vi "Create Server.vi"(5 "Server Key File (.key)":path, 7 "Server Certificate File (.crt)":path, 8 "error in":errorcluster, 11 "Server Address":string) -> (0 "error out":errorcluster, 3 "gRPC server out":refnum<class "Servicer.lvclass">)   [LabVIEW 2019, in "gRPC-servicer.lvlib" / "Servicer.lvclass"]
uses:
  Servicer.lvclass
  gRPC lv Support/grpc-lvsupport.lvlib
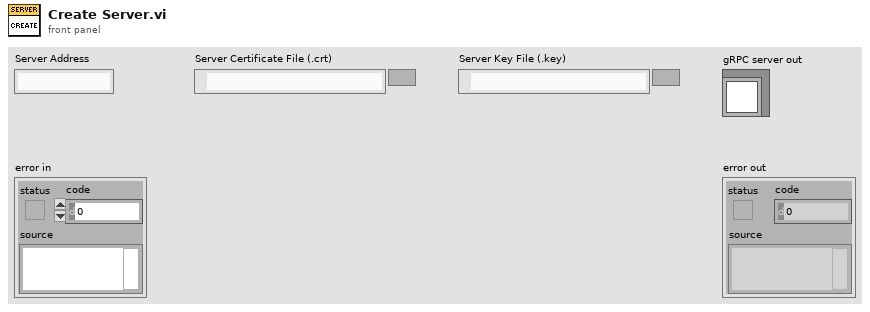
[diagram p1: front panel]
types:
  T1 = typedef "grpc-lvsupport.lvlib/grpcId.ctl" = u64
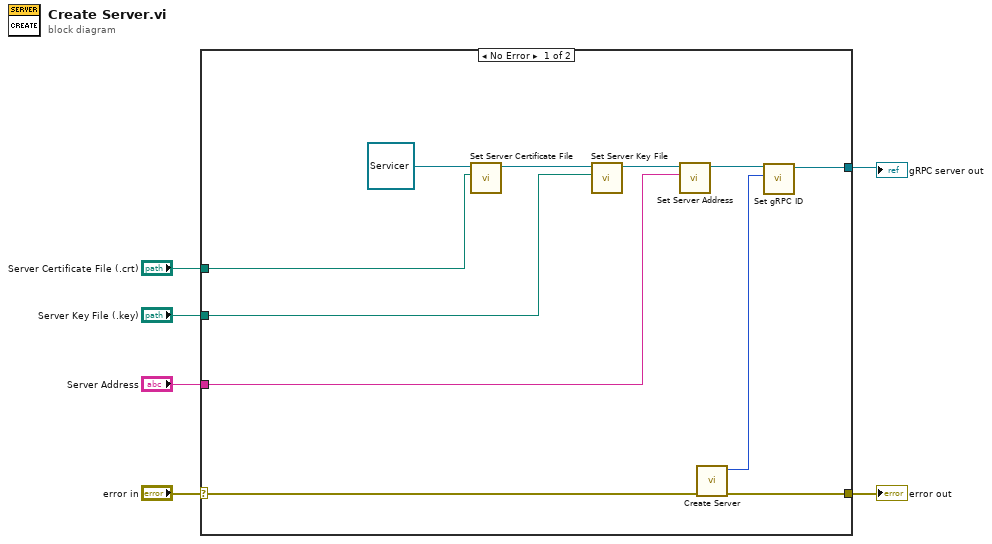
[diagram p0: block diagram]
diagram:
  n1 = case shown="No Error" "error in" {
    selector: "error in" -> [w17 w18]
    tunnel: [w16 w18] -> w5
    tunnel: [w7 _] -> w4
    tunnel: "Server Certificate File (.crt)" -> [w11 _]
    tunnel: "Server Key File (.key)" -> [w10 _]
    tunnel: "Server Address" -> [w9 _]
    frame No Error {
      n2 = call "Set Server Certificate File.vi"("Server Certificate File (.crt)"=w11, "gRPC server in"=refnum<class "Servicer.lvclass"> refnum ("OOP Server out")) -> ("gRPC server out"=w14:refnum<class "Servicer.lvclass">)  [unwired: 9 in]
      n3 = call "Set Server Key File.vi"("Server Key File (.key)"=w10, "gRPC server in"=w14) -> ("gRPC server out"=w13:refnum<class "Servicer.lvclass">)  [unwired: 9 in]
      n4 = call "Set Server Address.vi"("Server Address"=w9, "gRPC server in"=w13) -> ("gRPC server out"=w12:refnum<class "Servicer.lvclass">)  [unwired: 9 in]
      n5 = call "Create Server.vi"("error in"=w17) -> ("error out"=w16:errorcluster, "gRPCid out"=w8:T1)  [unwired: 9 in]
      n6 = call "Set gRPC ID.vi"("gRPC ID"=w8, "gRPC server in"=w12) -> ("gRPC server out"=w7:refnum<class "Servicer.lvclass">)  [unwired: 9 in]
    }
    frame Error {
    }
  }
  "error out" <- w5
  "gRPC server out" <- w4
